vi "Write Post-Measurement Settling Duration.vi"(8 "error in (no error)":errorcluster, 10 "post-measurement settling duration [s]":dbl, 11 "signal configuration":refnum<class "SV Signal.lvclass">) -> (0 "error out":errorcluster, 3 "signal configuration":refnum<class "SV Signal.lvclass">)   [LabVIEW 2017, in "SV Signal.lvclass"]
uses:
  <vilib>/addons/_NISVFA/_Generation/Signal Generation/SV Signal/SV Signal.lvclass
  <vilib>/addons/_NISVFA/_Generation/Signal Generation/SV Signal/SV Signal.lvclass/SV Signal.ctl
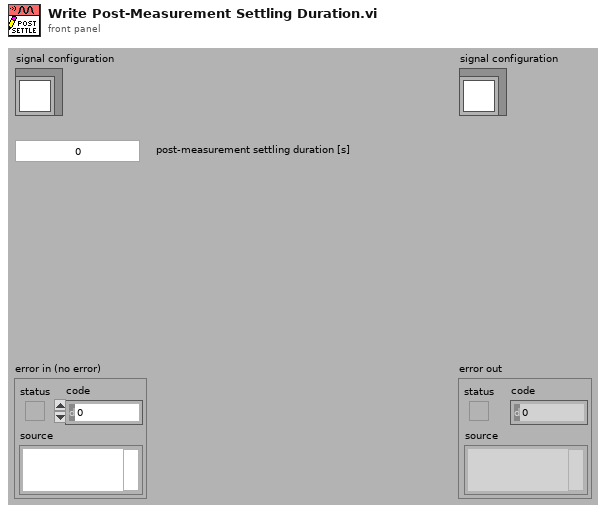
[diagram p1: front panel]
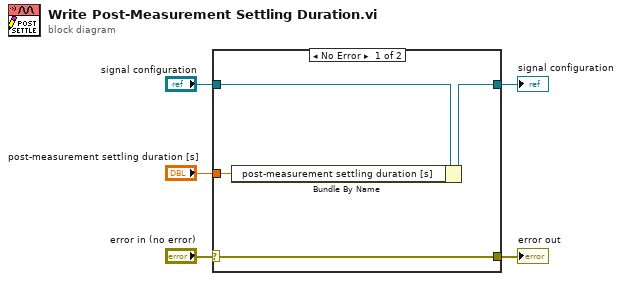
[diagram p0: block diagram]
diagram:
  n1 = case shown="No Error" "error in (no error)" {
    selector: "error in (no error)" -> [w9 w10]
    tunnel: [w9 w10] -> w4
    tunnel: [w7 w11] -> w2
    tunnel: "signal configuration" -> [w8 w11]
    tunnel: "post-measurement settling duration [s]" -> [w6 _]
    frame No Error {
      n2 = Bundle By Name(cluster=w8, "post-measurement settling duration [s]"=w6) -> (w7:refnum<class "SV Signal.lvclass">)
    }
    frame Error {
    }
  }
  "error out" <- w4
  "signal configuration" <- w2
